vi "DiscArchiver.ProcCases.vi"(0 "i ref in":refnum<vi>, 1 "selector":string, 2 "Data":T1, 3 "call cluster":T2={"Object"="", "Selector"="", "CallType"=enum."synchronous", "Async Object"="", "Async Selector"="", "Data Descriptor"="", "Data"=[], "Error #"=0, "Expire"=0}, 5 "error in (no error)":errorcluster) -> (14 "i ref out":refnum<vi>, 17 "answer cluster":T2={"Object"="", "Selector"="", "CallType"=enum."synchronous", "Async Object"="", "Async Selector"="", "Data Descriptor"="", "Data"=[], "Error #"=0, "Expire"=0}, 19 "error out":errorcluster)   [LabVIEW 2014, in "DiscArchiver.lvlib"]
doc: "This method is called by a process from within the default case in the event loop. The methods of a class that are linked to events will be called from THIS method. Add your code here."
uses:
  DiscArchiver.lvlib
  CSCore/CSSystem/CoreDefs/CoreDefs.call_type.ctl
  CSCore/BaseProcess/BaseProcess.descriptor string definition.ctl
  CSCore/CSSystem/CoreDefs/CoreDefs.rawDataType.ctl
  CSCore/CSSystem/CoreLib/CoreLib.string 2 byte array.vi
  CSCore/CSSystem/CoreLib/CoreLib.byte array 2 string.vi
  CSCore/CSSystem/CoreLib/CoreLib.int 2 byte array.vi
  CSCore/CSSystem/CoreLib/CoreLib.byte array 2 short.vi
  CSCore/BaseProcess/BaseProcess.lvlib
  CSCore/CSSystem/CoreLib/CoreLib.lvlib
  CSCore/CAEObj/CAEObj.lvlib
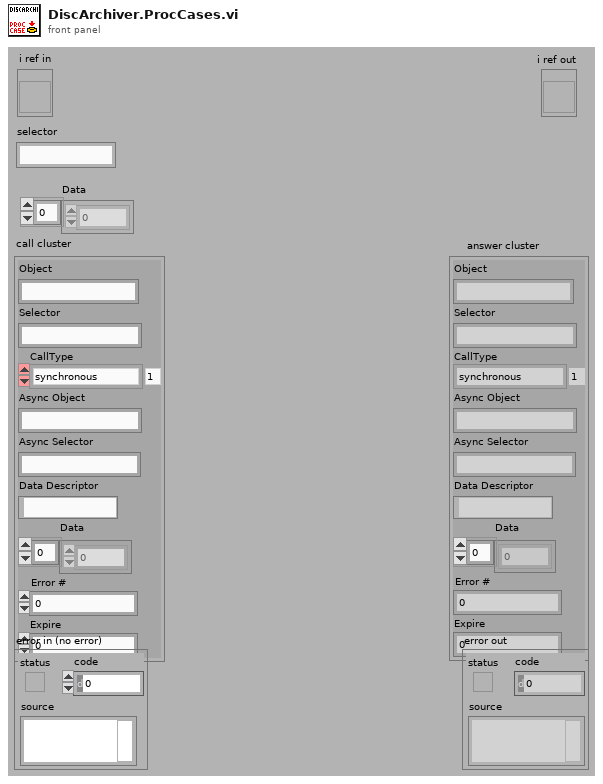
[diagram p1: front panel]
types:
  T1 = typedef "CoreDefs.rawDataType.ctl" = i8[]
  T2 = typedef "CoreDefs.call_type.ctl" = cluster{"Object":string, "Selector":string, "CallType":enum16{"simple", "synchronous", "asynchronous"}, "Async Object":string, "Async Selector":string, "Data Descriptor":T3, "Data":T1, "Error #":i32, "Expire":u32}
  T3 = typedef "BaseProcess.lvlib/BaseProcess.descriptor string definition.ctl" = string
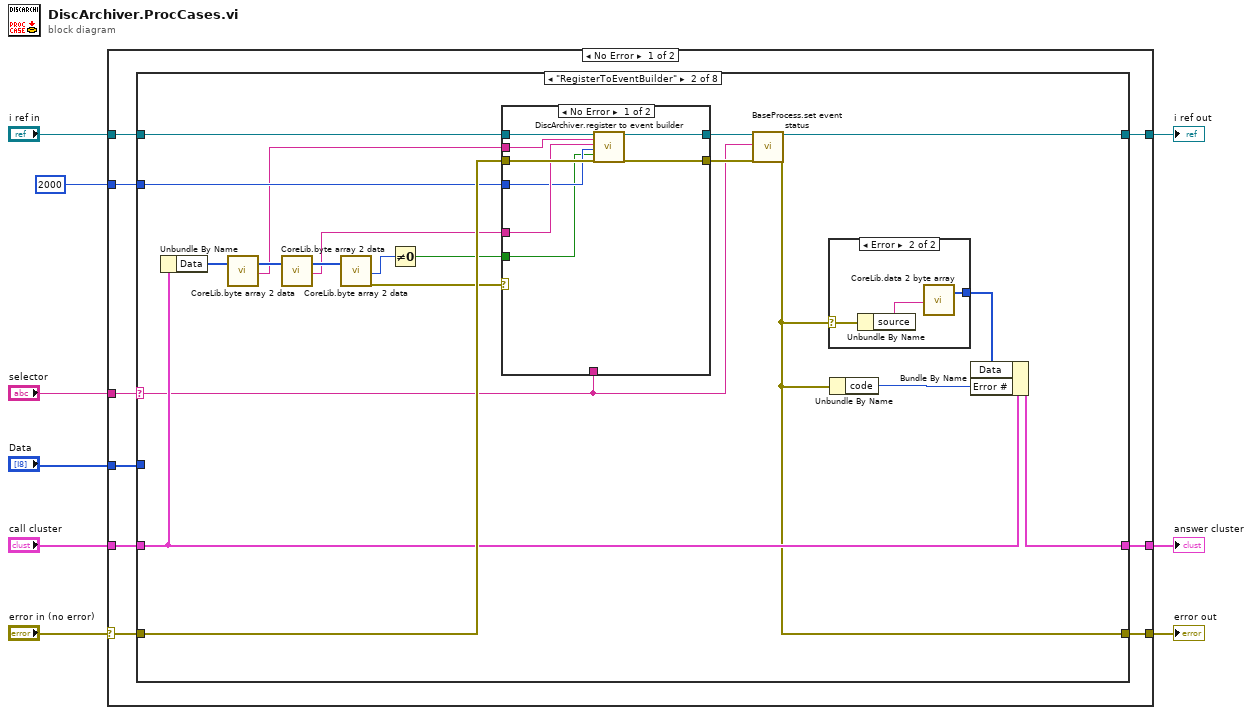
[diagram p0: block diagram]
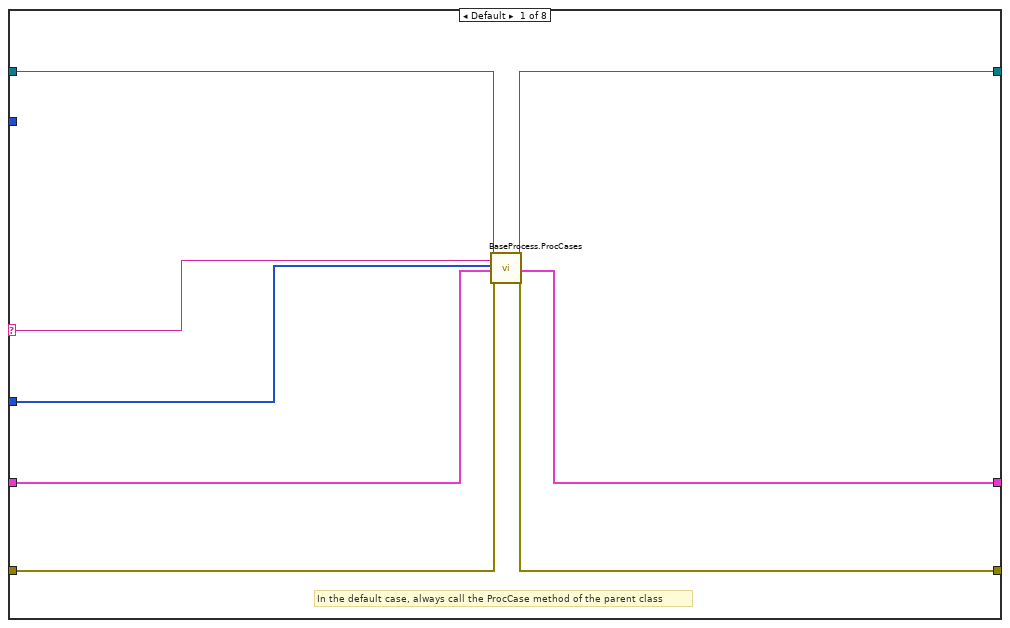
[diagram p2: hidden frame]
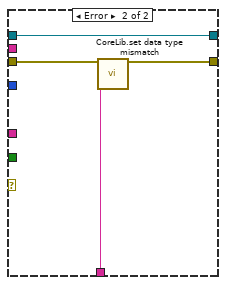
[diagram p4: hidden frame]
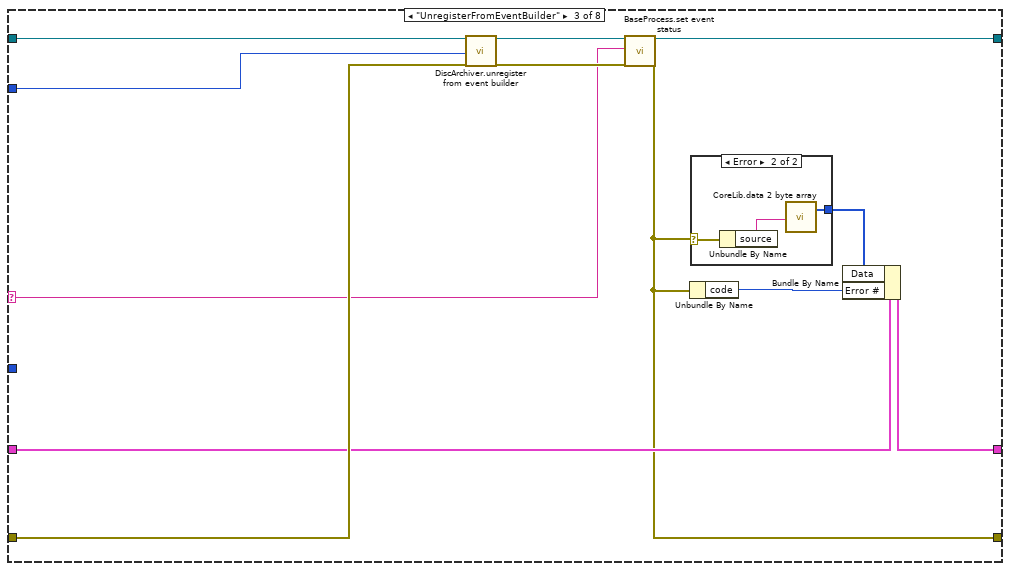
[diagram p5: hidden frame]
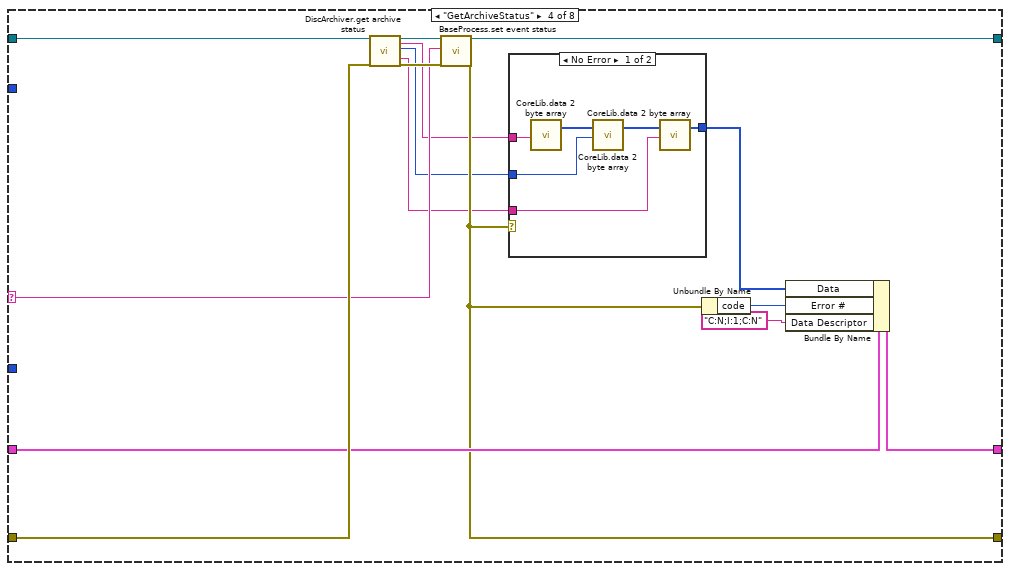
[diagram p7: hidden frame]
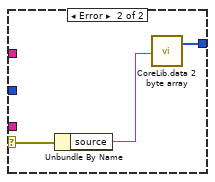
[diagram p8: hidden frame]
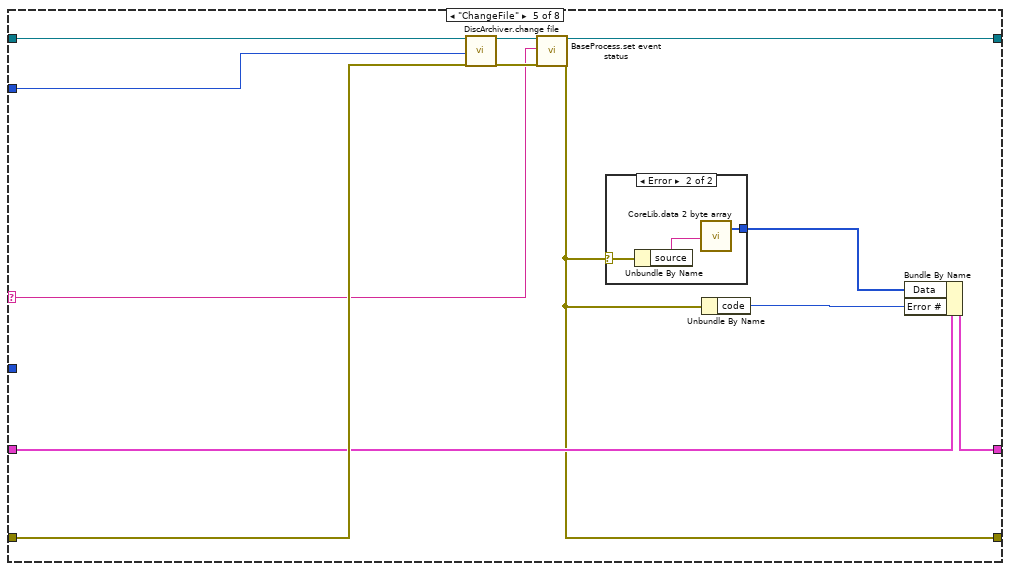
[diagram p9: hidden frame]
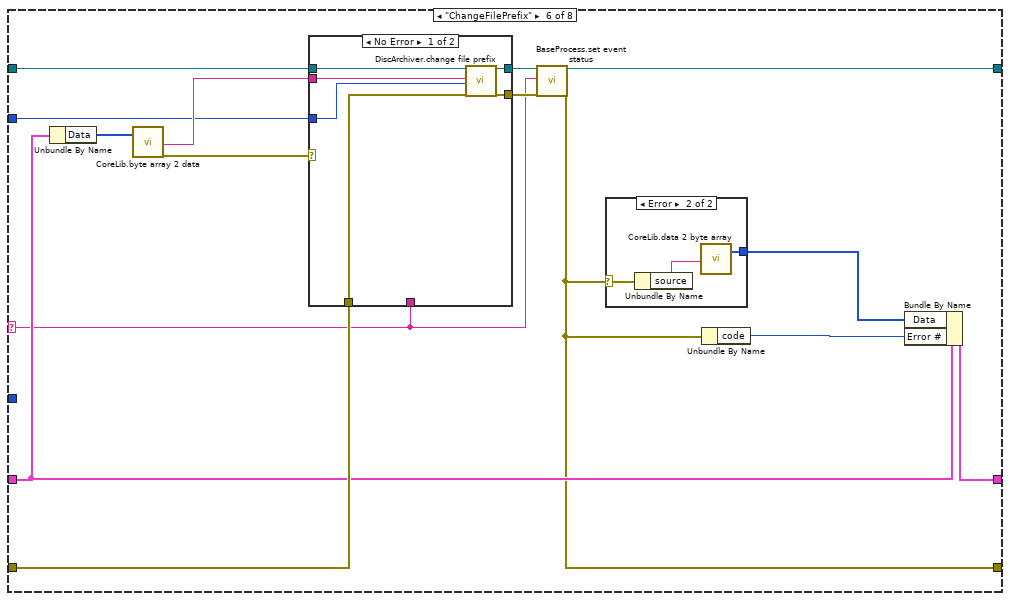
[diagram p11: hidden frame]
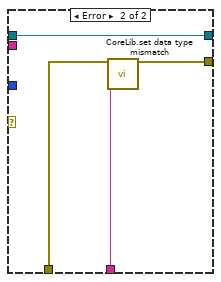
[diagram p13: hidden frame]
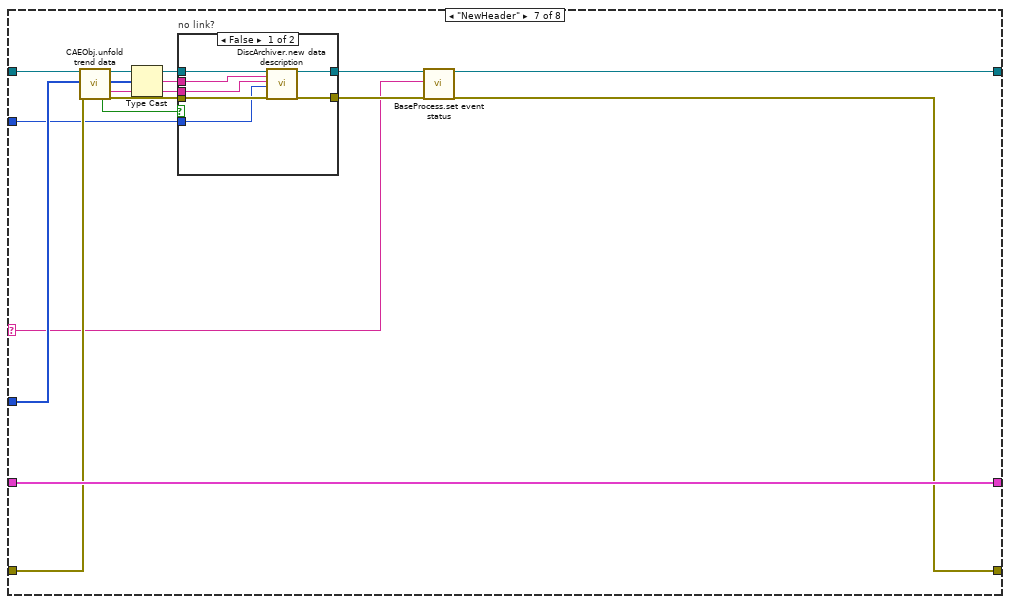
[diagram p14: hidden frame]
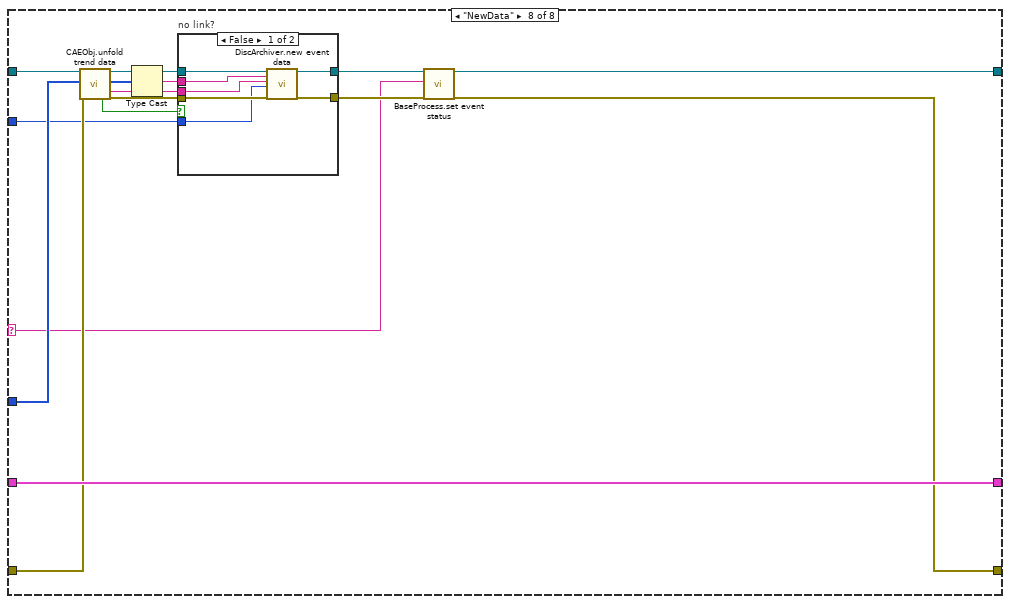
[diagram p16: hidden frame]
diagram:
  n1 = case shown="No Error" "error in (no error)" {
    selector: "error in (no error)" -> [w10 w196]
    tunnel: "selector" -> [w18 _]
    tunnel: [w17 w195] -> w8
    tunnel: "Data" -> [w16 _]
    tunnel: "call cluster" -> [w15 w195]
    tunnel: "i ref in" -> [w14 w194]
    tunnel: [w13 w194] -> w4
    tunnel: [w12 w196] -> w3
    tunnel: 2000 ("ms timeout (100)") -> [w11 _]
    frame No Error {
      n2 = case shown="\"RegisterToEventBuilder\"" w18 {
        selector: w18 -> [w20 w37 w66 w83 w105 w122 w146 w171]
        tunnel: w16 -> [w21 _ _ _ _ _ w158 w183]
        tunnel: w14 -> [w19 w46 w73 w91 w112 w130 w153 w178]
        tunnel: [w26 w36 w65 w82 w106 w124 w145 w170] -> w13
        tunnel: w15 -> [w22 w43 w70 w88 w104 w123 w159 w184]
        tunnel: [w23 w42 w69 w87 w109 w127 w159 w184] -> w17
        tunnel: w10 -> [w25 w45 w72 w90 w111 w129 w154 w179]
        tunnel: [w24 w38 w63 w84 w102 w121 w144 w169] -> w12
        tunnel: w11 -> [_ w35 w64 _ w103 w117 w149 w174]
        frame Default {
          # "In the default case, always call the ProcCase method of the parent class"
          n3 = call "BaseProcess.ProcCases.vi"("i ref in"=w19, "selector"=w20, "Data"=w21, "call cluster"=w22, "error in (no error)"=w25) -> ("i ref out"=w26:refnum<vi>, "answer cluster"=w23:T2, "error out"=w24:errorcluster)  [unwired: 12 in]
        }
        frame "RegisterToEventBuilder" {
          n4 = Unbundle By Name(w43) -> ("Data"=w34:T1)
          n5 = call-poly "CoreLib.byte array 2 data.vi"("byteArray"=w34) -> ("byteArray out"=w33:T1, "string"=w31:string)  [unwired: 16 in, 1 out]
          n6 = call-poly "CoreLib.byte array 2 data.vi"("byteArray"=w33) -> ("byteArray out"=w32:T1, "string"=w30:string)  [unwired: 16 in, 1 out]
          n7 = call-poly "CoreLib.byte array 2 data.vi"("byteArray"=w32) -> ("i16"=w29:i16, "error out"=w27:errorcluster)  [unwired: 16 in, 1 out]
          n8 = Not Equal To 0?(x=w29) -> (x != 0?=w28:bool)
          n9 = case shown="No Error" w27 {
            tunnel: [w56 w61] -> w40
            tunnel: w46 -> [w57 w61]
            tunnel: w45 -> [w55 w60]
            tunnel: [w54 w59] -> w39
            tunnel: w30 -> [w52 _]
            tunnel: w37 -> [_ w58]
            tunnel: w31 -> [w53 _]
            tunnel: w35 -> [w51 _]
            tunnel: w28 -> [w50 _]
            frame No Error {
              n10 = call "DiscArchiver.register to event builder.vi"("i ref in"=w57, "collector"=w53, "filePrefix"=w52, "ms timeout (10000)"=w51, "complete"=w50, "error in (no error)"=w55) -> ("i ref out"=w56:refnum<vi>, "error out"=w54:errorcluster)  [unwired: 11 in, 1 out]
            }
            frame Error {
              n11 = call "CoreLib.set data type mismatch.vi"("error in (no error)"=w60, "error source"=w58) -> ("error out"=w59:errorcluster)  [unwired: 17 in]
            }
          }
          n12 = call "BaseProcess.set event status.vi"("i ref in"=w40, "EventStatus"=w37, "error in (no error)"=w39) -> ("i ref out"=w36:refnum<vi>, "error out"=w38:errorcluster)  [unwired: 14 in, 1 out]
          n13 = case shown="Error" w38 {
            selector: w38 -> [_ w49]
            tunnel: [_ w47] -> w41
            frame No Error {
            }
            frame Error {
              n14 = Unbundle By Name(w49) -> ("source"=w48:string)
              n15 = call-poly "CoreLib.data 2 byte array.vi"("string"=w48) -> ("byteArray out"=w47:T1)  [unwired: 18 in]
            }
          }
          n16 = Unbundle By Name(w38) -> ("code"=w44:i32)
          n17 = Bundle By Name(cluster=w43, "Data"=w41, "Error #"=w44) -> (w42:T2)
        }
        frame "UnregisterFromEventBuilder" {
          n18 = call "DiscArchiver.unregister from event builder.vi"("i ref in"=w73, "ms timeout (10000)"=w64, "error in (no error)"=w72) -> ("i ref out"=w68:refnum<vi>, "error out"=w67:errorcluster)  [unwired: 14 in, 1 out]
          n19 = call "BaseProcess.set event status.vi"("i ref in"=w68, "EventStatus"=w66, "error in (no error)"=w67) -> ("i ref out"=w65:refnum<vi>, "error out"=w63:errorcluster)  [unwired: 14 in, 1 out]
          n20 = Unbundle By Name(w63) -> ("code"=w71:i32)
          n21 = case shown="Error" w63 {
            selector: w63 -> [_ w76]
            tunnel: [_ w74] -> w62
            frame No Error {
            }
            frame Error {
              n22 = Unbundle By Name(w76) -> ("source"=w75:string)
              n23 = call-poly "CoreLib.data 2 byte array.vi"("string"=w75) -> ("byteArray out"=w74:T1)  [unwired: 18 in]
            }
          }
          n24 = Bundle By Name(cluster=w70, "Data"=w62, "Error #"=w71) -> (w69:T2)
        }
        frame "GetArchiveStatus" {
          n25 = call "DiscArchiver.get archive status.vi"("i ref in"=w91, "error in (no error)"=w90) -> ("i ref out"=w86:refnum<vi>, "actual file"=w81:string, "# of items"=w80:i32, "eventBuilder"=w79:string, "error out"=w85:errorcluster)  [unwired: 13 in]
          n26 = call "BaseProcess.set event status.vi"("i ref in"=w86, "EventStatus"=w83, "error in (no error)"=w85) -> ("i ref out"=w82:refnum<vi>, "error out"=w84:errorcluster)  [unwired: 14 in, 1 out]
          n27 = case shown="No Error" w84 {
            selector: w84 -> [_ w100]
            tunnel: w81 -> [w97 _]
            tunnel: w80 -> [w96 _]
            tunnel: w79 -> [w93 _]
            tunnel: [w92 w98] -> w78
            frame No Error {
              n28 = call-poly "CoreLib.data 2 byte array.vi"("string"=w97) -> ("byteArray out"=w95:T1)  [unwired: 18 in]
              n29 = call-poly "CoreLib.data 2 byte array.vi"("byteArray"=w95, "i32"=w96) -> ("byteArray out"=w94:T1)  [unwired: 17 in]
              n30 = call-poly "CoreLib.data 2 byte array.vi"("byteArray"=w94, "string"=w93) -> ("byteArray out"=w92:T1)  [unwired: 17 in]
            }
            frame Error {
              n31 = Unbundle By Name(w100) -> ("source"=w99:string)
              n32 = call-poly "CoreLib.data 2 byte array.vi"("string"=w99) -> ("byteArray out"=w98:T1)  [unwired: 18 in]
            }
          }
          n33 = Unbundle By Name(w84) -> ("code"=w89:i32)
          n34 = Bundle By Name(cluster=w88, "Data"=w78, "Error #"=w89, "Data Descriptor"="C:N;I:1;C:N" ("source")) -> (w87:T2)
        }
        frame "ChangeFile" {
          n35 = call "DiscArchiver.change file.vi"("i ref in"=w112, "ms timeout (10000)"=w103, "error in (no error)"=w111) -> ("i ref out"=w108:refnum<vi>, "error out"=w107:errorcluster)  [unwired: 14 in, 1 out]
          n36 = call "BaseProcess.set event status.vi"("i ref in"=w108, "EventStatus"=w105, "error in (no error)"=w107) -> ("i ref out"=w106:refnum<vi>, "error out"=w102:errorcluster)  [unwired: 14 in, 1 out]
          n37 = case shown="Error" w102 {
            selector: w102 -> [_ w115]
            tunnel: [_ w113] -> w101
            frame No Error {
            }
            frame Error {
              n38 = Unbundle By Name(w115) -> ("source"=w114:string)
              n39 = call-poly "CoreLib.data 2 byte array.vi"("string"=w114) -> ("byteArray out"=w113:T1)  [unwired: 18 in]
            }
          }
          n40 = Unbundle By Name(w102) -> ("code"=w110:i32)
          n41 = Bundle By Name(cluster=w104, "Data"=w101, "Error #"=w110) -> (w109:T2)
        }
        frame "ChangeFilePrefix" {
          n42 = Unbundle By Name(w123) -> ("Data"=w119:T1)
          n43 = call-poly "CoreLib.byte array 2 data.vi"("byteArray"=w119) -> ("string"=w118:string, "error out"=w116:errorcluster)  [unwired: 16 in, 1 out]
          n44 = case shown="No Error" w116 {
            tunnel: w130 -> [w139 w143]
            tunnel: w129 -> [w138 w141]
            tunnel: [w137 w143] -> w126
            tunnel: [w136 w142] -> w125
            tunnel: w118 -> [w135 _]
            tunnel: w122 -> [_ w140]
            tunnel: w117 -> [w134 _]
            frame No Error {
              n45 = call "DiscArchiver.change file prefix.vi"("i ref in"=w139, "file prefix"=w135, "ms timeout (10000)"=w134, "error in (no error)"=w138) -> ("i ref out"=w137:refnum<vi>, "error out"=w136:errorcluster)  [unwired: 13 in, 1 out]
            }
            frame Error {
              n46 = call "CoreLib.set data type mismatch.vi"("error in (no error)"=w141, "error source"=w140) -> ("error out"=w142:errorcluster)  [unwired: 17 in]
            }
          }
          n47 = call "BaseProcess.set event status.vi"("i ref in"=w126, "EventStatus"=w122, "error in (no error)"=w125) -> ("i ref out"=w124:refnum<vi>, "error out"=w121:errorcluster)  [unwired: 14 in, 1 out]
          n48 = case shown="Error" w121 {
            selector: w121 -> [_ w133]
            tunnel: [_ w131] -> w120
            frame No Error {
            }
            frame Error {
              n49 = Unbundle By Name(w133) -> ("source"=w132:string)
              n50 = call-poly "CoreLib.data 2 byte array.vi"("string"=w132) -> ("byteArray out"=w131:T1)  [unwired: 18 in]
            }
          }
          n51 = Unbundle By Name(w121) -> ("code"=w128:i32)
          n52 = Bundle By Name(cluster=w123, "Data"=w120, "Error #"=w128) -> (w127:T2)
        }
        frame "NewHeader" {
          n53 = call "CAEObj.unfold trend data.vi"("i ref in"=w153, "raw trend data"=w158, "error in (no error)"=w154) -> ("no link"=w157:bool, "i ref out"=w152:refnum<vi>, "data"=w156:i8[], "typeDescriptor"=w150:string, "error out"=w151:errorcluster)  [unwired: 8 in, 4 out]
          n54 = Type Cast(x=w156) -> (*(type *) &x=w155:string)  [unwired: 1 in]
          n55 = case "no link?" shown="False" w157 {
            tunnel: [w161 w168] -> w148
            tunnel: w152 -> [w165 w168]
            tunnel: w155 -> [w164 _]
            tunnel: w151 -> [w166 w167]
            tunnel: w150 -> [w163 _]
            tunnel: w149 -> [w162 _]
            tunnel: [w160 w167] -> w147
            frame False {
              n56 = call "DiscArchiver.new data description.vi"("i ref"=w165, "dataDescription"=w164, "descriptor"=w163, "ms timeout (10000)"=w162, "error in (no error)"=w166) -> ("i ref out"=w161:refnum<vi>, "error out"=w160:errorcluster)  [unwired: 12 in, 1 out]
            }
            frame True {
            }
          }
          n57 = call "BaseProcess.set event status.vi"("i ref in"=w148, "EventStatus"=w146, "error in (no error)"=w147) -> ("i ref out"=w145:refnum<vi>, "error out"=w144:errorcluster)  [unwired: 14 in, 1 out]
        }
        frame "NewData" {
          n58 = call "CAEObj.unfold trend data.vi"("i ref in"=w178, "raw trend data"=w183, "error in (no error)"=w179) -> ("no link"=w182:bool, "i ref out"=w177:refnum<vi>, "data"=w181:i8[], "typeDescriptor"=w175:string, "error out"=w176:errorcluster)  [unwired: 8 in, 4 out]
          n59 = Type Cast(x=w181) -> (*(type *) &x=w180:string)  [unwired: 1 in]
          n60 = case "no link?" shown="False" w182 {
            tunnel: [w186 w193] -> w173
            tunnel: w177 -> [w190 w193]
            tunnel: w180 -> [w189 _]
            tunnel: w176 -> [w191 w192]
            tunnel: w175 -> [w188 _]
            tunnel: w174 -> [w187 _]
            tunnel: [w185 w192] -> w172
            frame False {
              n61 = call "DiscArchiver.new event data.vi"("i ref"=w190, "eventData"=w189, "descriptor"=w188, "ms timeout (10000)"=w187, "error in (no error)"=w191) -> ("i ref out"=w186:refnum<vi>, "error out"=w185:errorcluster)  [unwired: 12 in, 1 out]
            }
            frame True {
            }
          }
          n62 = call "BaseProcess.set event status.vi"("i ref in"=w173, "EventStatus"=w171, "error in (no error)"=w172) -> ("i ref out"=w170:refnum<vi>, "error out"=w169:errorcluster)  [unwired: 14 in, 1 out]
        }
      }
    }
    frame Error {
    }
  }
  "answer cluster" <- w8
  "i ref out" <- w4
  "error out" <- w3
